vi "writeSDOI16.vi"(6 "object sub-index (0)":u8 format="%x", 7 "object index":u16 format="%x", 8 "error in (no error)":errorcluster, 9 "interface object in":refnum<k20>, 10 "inputNumber":i16, 11 "MotorControllerClass in":refnum<class "MotorControllerClass.lvclass">) -> (0 "error out":errorcluster, 1 "interface object out":refnum<k20>, 2 "completion code":u32, 3 "MotorControllerClass out":refnum<class "MotorControllerClass.lvclass">)   [LabVIEW 2018, in "MotorControllerClass.lvclass"]
uses:
  BMS/MotorControllerClass.lvclass
  <vilib>/CANopenLib/CANOPEN.llb/CANopen SDO Create.vi
  <vilib>/CANopenLib/CANOPEN.llb/CANopen SDO Write [I16].vi
  <vilib>/CANopenLib/CANOPEN.llb/CANopen SDO Close.vi
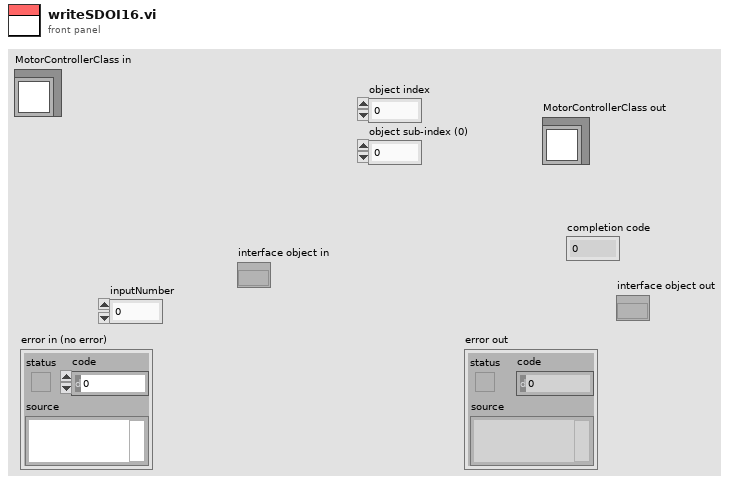
[diagram p1: front panel]
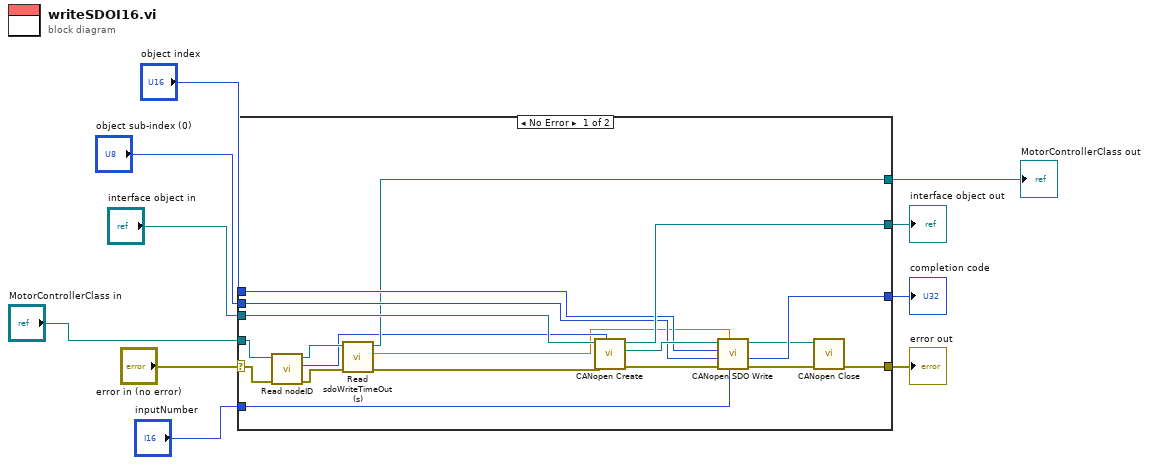
[diagram p0: block diagram]
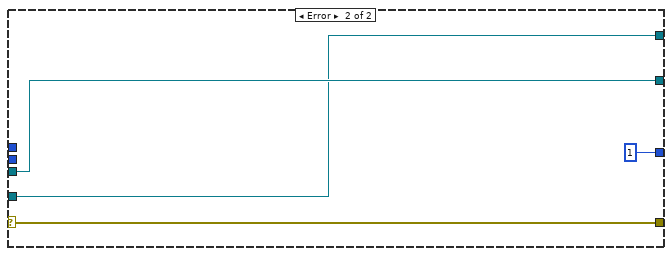
[diagram p2: hidden frame]
diagram:
  n1 = case shown="No Error" "error in (no error)" {
    selector: "error in (no error)" -> [w14 w33]
    tunnel: [w22 w33] -> w3
    tunnel: [w29 w31] -> w8
    tunnel: "interface object in" -> [w28 w31]
    tunnel: "object index" -> [w26 _]
    tunnel: "object sub-index (0)" -> [w25 _]
    tunnel: [w24 u32 1 ("completion code")] -> w5
    tunnel: "inputNumber" -> [w19 _]
    tunnel: "MotorControllerClass in" -> [w17 w30]
    tunnel: [w16 w30] -> w1
    frame No Error {
      n2 = call-dynamic "Read nodeID.vi"("error in (no error)"=w14, "MotorControllerClass in"=w17) -> ("error out"=w13:errorcluster, "nodeID"=w15:u8, "MotorControllerClass out"=w18:refnum<class "MotorControllerClass.lvclass">)  [unwired: 7 in]
      n3 = call-dynamic "Read sdoWriteTimeOut(s).vi"("error in (no error)"=w13, "MotorControllerClass in"=w18) -> ("error out"=w12:errorcluster, "sdoWriteTimeOut(s)"=w11:dbl, "MotorControllerClass out"=w16:refnum<class "MotorControllerClass.lvclass">)  [unwired: 7 in]
      n4 = call-poly <vilib>:"CANopen Create.vi"("node-ID"=w15, "error in (no error)"=w12, "interface object in"=w28) -> ("error out"=w20:errorcluster, "SDO object out"=w27:refnum<k20>, "interface object out"=w29:refnum<k20>)  [unwired: 6 in]
      n5 = call-poly <vilib>:"CANopen SDO Write.vi"("I16 data"=w19, "timeout (1s)"=w11, "error in (no error)"=w20, "object sub-index (0)"=w25, "object index"=w26, "SDO object in"=w27) -> ("error out"=w23:errorcluster, "completion code"=w24:u32, "SDO object out"=w21:refnum<k20>)  [unwired: 3 in]
      n6 = call-poly <vilib>:"CANopen Close.vi"("error in (no error)"=w23, "SDO object in"=w21) -> ("error out"=w22:errorcluster)  [unwired: 9 in]
    }
    frame Error {
    }
  }
  "error out" <- w3
  "interface object out" <- w8
  "completion code" <- w5
  "MotorControllerClass out" <- w1
